vi "resonant.z.stack.run_MD.vi"() -> ()   [LabVIEW 2012]
uses:
  Custom Controls/experiment type.ctl
  GFG/GFGnumericGet.vi
  GFG/GFGfpRefGet.vi
  GFG/GFGbooleanGet.vi
  GFG/GFG library.lvlib
panel:
  out "x-y":u32
  out "error out 2":errorcluster
  out "transposed array":dbl[][](array[numeric])
  out "data":dbl[][](array[numeric])
  in  "error in (no error)":errorcluster
  out "error out":errorcluster
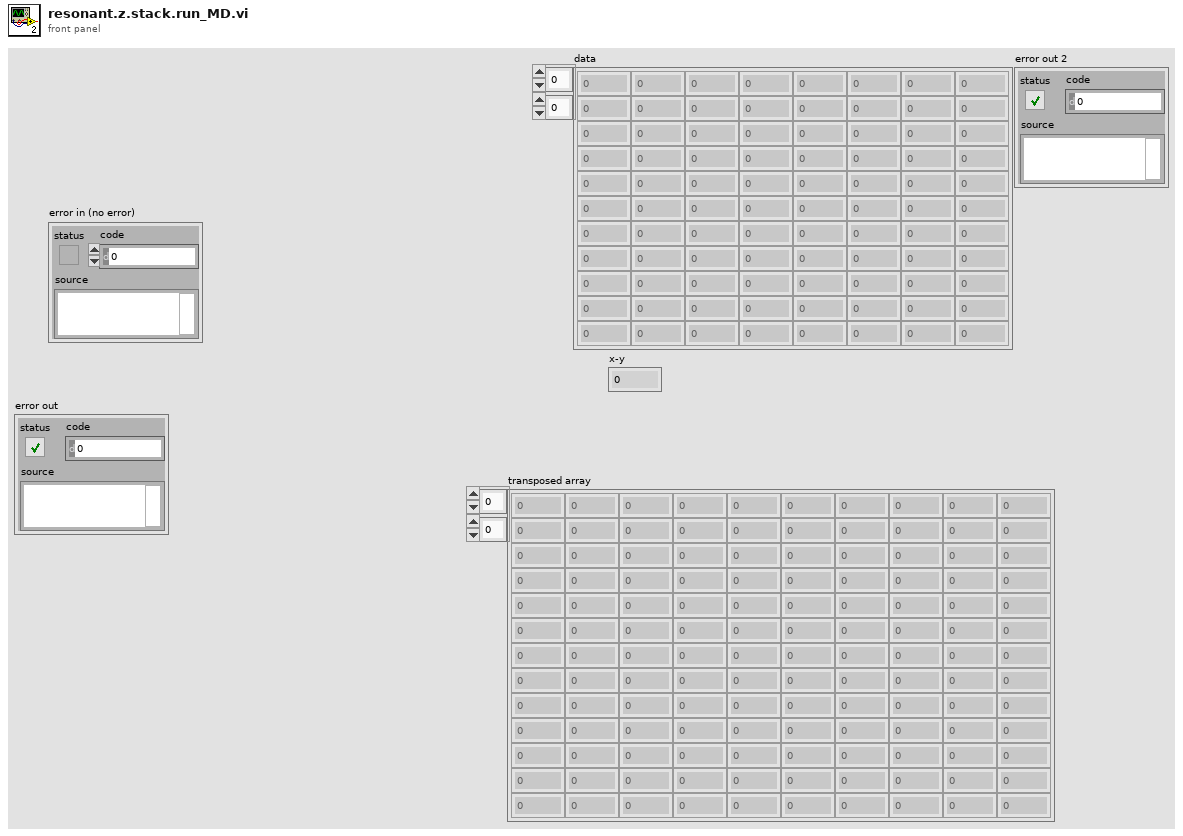
[diagram p1: front panel]
types:
  T1 = typedef "experiment type.ctl" = string
  T2 = enum8{"Enabled", "Disabled", "Disabled and Grayed Out"}
  T3 = cluster{"WaveformChartRef":refnum<vi>, "DigitalRef":refnum<vi>, "ArrayRef":refnum<vi>, "TabControlRef":refnum<vi>, "EnumRef":refnum<vi>, "RingRef":refnum<vi>, "BooleanRef":refnum<vi>, "KnobRef":refnum<vi>, "SlideRef":refnum<vi>, "PathRef":refnum<vi>, "StringRef":refnum<vi>, "ComboBox":refnum<vi>, "WaveformGraphRef":refnum<vi>}
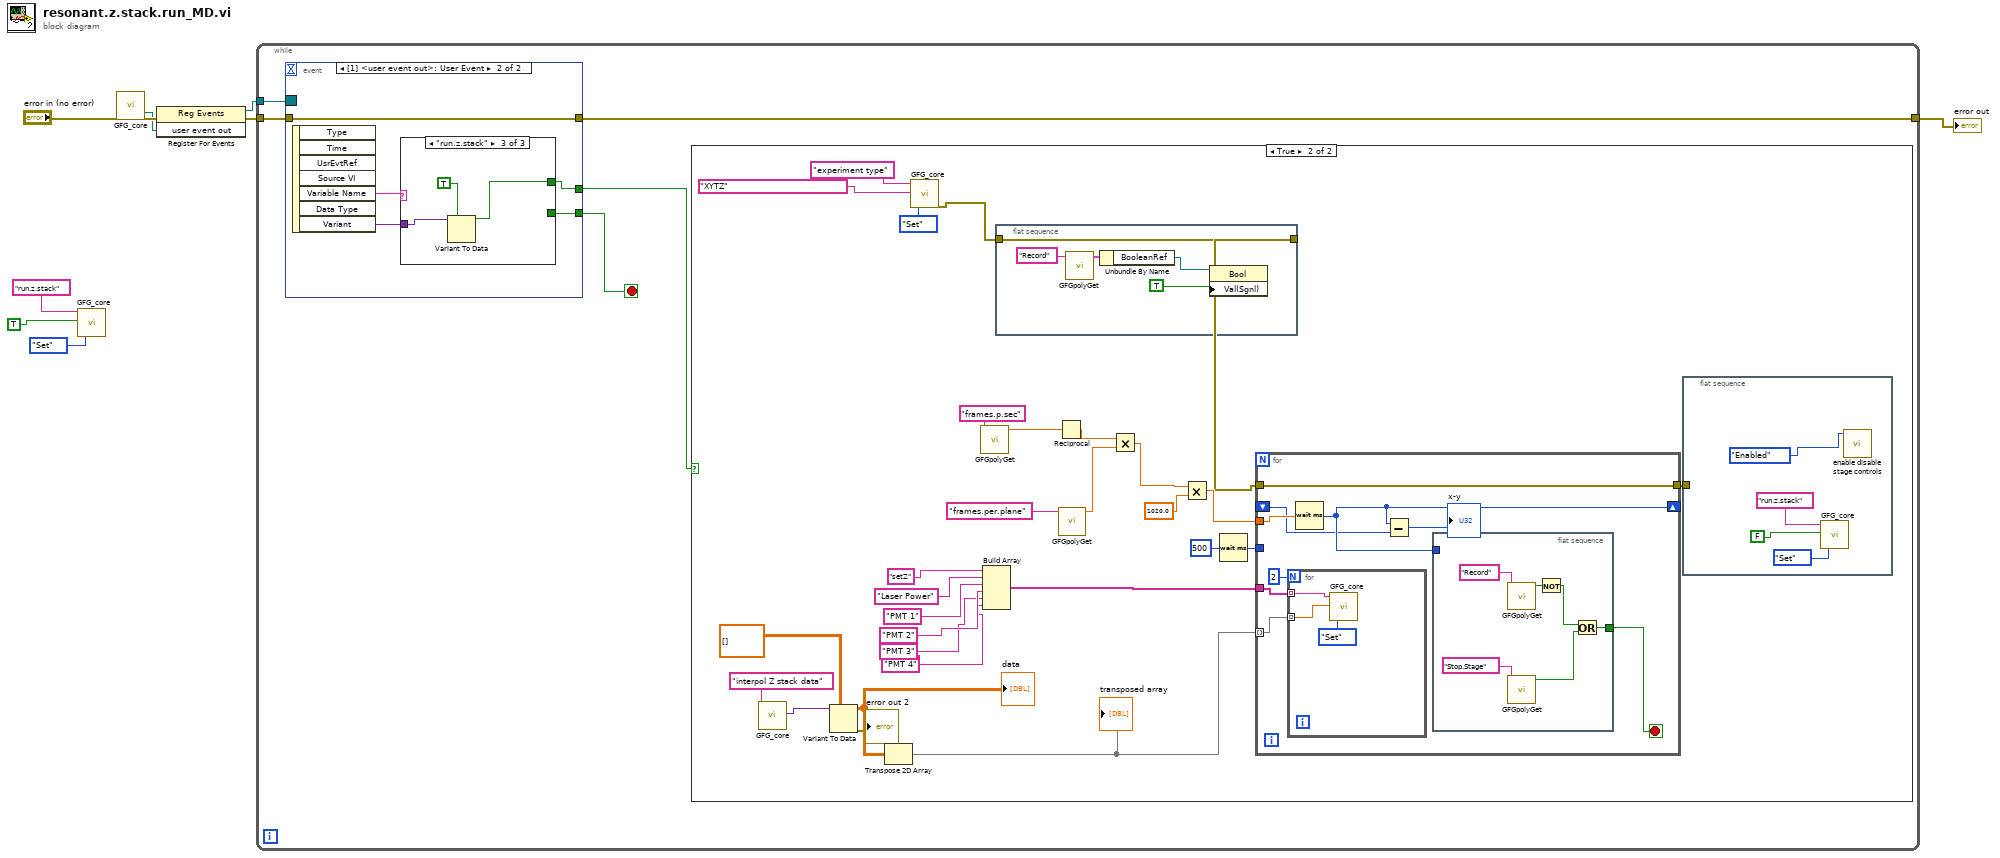
[diagram p0: block diagram]
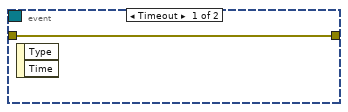
[diagram p3: hidden frame]
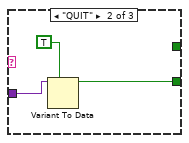
[diagram p5: hidden frame]
diagram:
  n1 = call "GFG_core.vi"("Variable Name in"="run.z.stack", "Variant in"=TRUE, "Action"=enum16{"Init", "Set", "Get"}."Set") -> ()  [unwired: 10 in, 7 out]
  n2 = call "GFG_core.vi"("error in (no error)"="error in (no error)") -> ("user event out"=w5:refnum<user-event>, "error out"=w6:errorcluster)  [unwired: 12 in, 5 out]
  n3 = register-events(error in=w6, w5) -> (reference out=w4:refnum<event-registration>, error out=w8:errorcluster)  [unwired: 1 in]
  n4 = while {
    tunnel: w4 -> [w14]
    tunnel: w8 -> [w13]
    tunnel: [w12] -> w9
    stop <- w11 stop-if-true
    n5 = event shown="[1] <user event out>: User Event" {
      selector: w14 -> [_ _]
      dyn-events: _ -> [_ _]
      timeout: _ -> [_ _]
      tunnel: w13 -> [w71 w76]
      tunnel: [w71 w76] -> w12
      tunnel: [_ w73] -> w11
      tunnel: [_ w72] -> w10
      event Timeout {
        n6 = event-data() -> ()  [unwired: 1 in, 2 out]
      }
      event User Event {
        n7 = event-data() -> ("Variable Name"=w75:string, "Variant"=w74:variant)  [unwired: 1 in, 5 out]
        n8 = case shown="\"run.z.stack\"" w75 {
          tunnel: w74 -> [_ w78 w81]
          tunnel: [_ w77 _] -> w73
          tunnel: [_ _ w80] -> w72
          frame "False", Default {
          }
          frame "QUIT" {
            n9 = Variant To Data(type=TRUE, Variant=w78) -> (data=w77:bool)  [unwired: 1 in, 1 out]
          }
          frame "run.z.stack" {
            n10 = Variant To Data(type=TRUE, Variant=w81) -> (data=w80:bool)  [unwired: 1 in, 1 out]
          }
        }
      }
    }
    n11 = case shown="True" w10 {
      frame False {
      }
      frame True {
        n12 = call "GFG_core.vi"("Variable Name in"="interpol Z stack data") -> ("Variant Out"=w37:variant)  [unwired: 12 in, 6 out]
        n13 = Variant To Data(type=dbl[][] [] ("Interpolated Data"), Variant=w37) -> (data=w35:dbl[][], error out=→"error out 2":errorcluster)  [unwired: 1 in]
        "data" <- w35
        n14 = Transpose 2D Array(2D array=w35) -> (transposed array=w34:dbl[][])
        "transposed array" <- w34
        n15 = call "GFG_core.vi"("Variable Name in"="experiment type", "Variant in"=T1 "XYTZ" ("experiment type"), "Action"=enum16{"Init", "Set", "Get"}."Set") -> ("error out"=w21:errorcluster)  [unwired: 10 in, 6 out]
        n16 = call-poly "GFGpolyGet.vi"("Variable Name in"="frames.p.sec") -> ("Numeric"=w42:dbl)  [unwired: 9 in, 1 out]
        n17 = Build Array("setZ" ("Variable Name in"), "Laser Power" ("Variable Name in"), "PMT 1" ("Variable Name in"), "PMT 2" ("Variable Name in"), "PMT 3" ("Variable Name in"), "PMT 4" ("Variable Name in")) -> (w27:string[])
        n18 = flat-sequence {
          tunnel: [w47] -> w22
          tunnel: w21 -> [w47]
          frame #0 {
            n19 = call-poly "GFGpolyGet.vi"("Variable Name in"="Record") -> ("output cluster"=w46:T3)  [unwired: 9 in, 1 out]
            n20 = Unbundle By Name(w46) -> ("BooleanRef"=w45:refnum<vi>)
            n21 = property class="Bool"(reference=w45, "Val(Sgnl)"=TRUE) -> ()  [unwired: 1 in, 2 out]
          }
        }
        n22 = Reciprocal(x=w42) -> (1/x=w19:dbl)
        n23 = call-poly "GFGpolyGet.vi"("Variable Name in"="frames.per.plane") -> ("Numeric"=w18:dbl)  [unwired: 9 in, 1 out]
        n24 = Multiply(x=w19, y=w18) -> (x*y=w17:dbl)
        n25 = Multiply(x=w17, y=1020.0) -> (x*y=w39:dbl)
        n26 = Wait (ms)(milliseconds to wait=u32 500) -> (millisecond timer value=w16:u32)
        n27 = for {
          tunnel: w39 -> [w61]
          tunnel: w34 -> [w60] mode=indexing
          tunnel: w27 -> [w59]
          tunnel: w22 -> [w57]
          tunnel: [w57] -> w23
          shift-right: [w56] -> _
          shift-left: _ -> [w55]
          tunnel: w16 -> [_]
          stop <- w58 stop-if-true
          n28 = for {
            N: 2 -> [_]
            tunnel: w60 -> [w69] mode=indexing
            tunnel: w59 -> [w70] mode=indexing
            n29 = call "GFG_core.vi"("Variable Name in"=w70, "Variant in"=w69, "Action"=enum16{"Init", "Set", "Get"}."Set") -> ()  [unwired: 10 in, 7 out]
          }
          n30 = Wait (ms)(milliseconds to wait=w61) -> (millisecond timer value=w56:u32)
          n31 = Subtract(x=w56, y=w55) -> (x-y=→"x-y":u32)
          n32 = flat-sequence {
            tunnel: w56 -> [_]
            tunnel: [w63] -> w58
            frame #0 {
              n33 = call-poly "GFGpolyGet.vi"("Variable Name in"="Record") -> ("Boolean"=w65:bool)  [unwired: 10 in]
              n34 = call-poly "GFGpolyGet.vi"("Variable Name in"="Stop.Stage") -> ("Boolean"=w64:bool)  [unwired: 10 in]
              n35 = Not(x=w65) -> (.not. x?=w62:bool)
              n36 = Or(x=w62, y=w64) -> (x .or. y?=w63:bool)
            }
          }
        }
        n37 = flat-sequence {
          tunnel: w23 -> [_]
          frame #0 {
            n38 = call "GFG_core.vi"("Variable Name in"="run.z.stack", "Variant in"=FALSE, "Action"=enum16{"Init", "Set", "Get"}."Set") -> ()  [unwired: 10 in, 7 out]
            n39 = call "enable disable stage controls.vi"("Disabled"=T2."Enabled") -> ()  [unwired: 11 in]
          }
        }
      }
    }
  }
  "error out" <- w9
